vi "ma_SML Data Packing (real input).vi"(6 "reset?":bool, 8 "error in (no error)":errorcluster, 9 "%overlap":dbl format="%.2f", 10 "size":i32, 11 "x":dbl[](array[numeric]) format="%.2f") -> (0 "error out":errorcluster, 1 "data ready?":bool, 3 "y":dbl[](array[numeric]) format="%.2f")   [LabVIEW 2020, in "NI_MAPro.lvlib"]
uses:
  NI_MAPro.lvlib
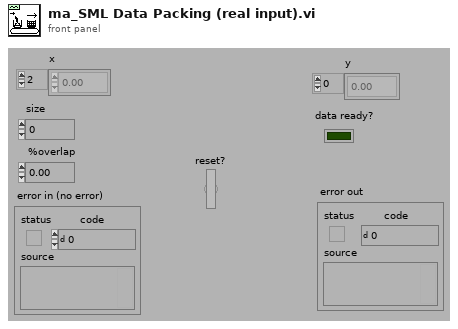
[diagram p1: front panel]
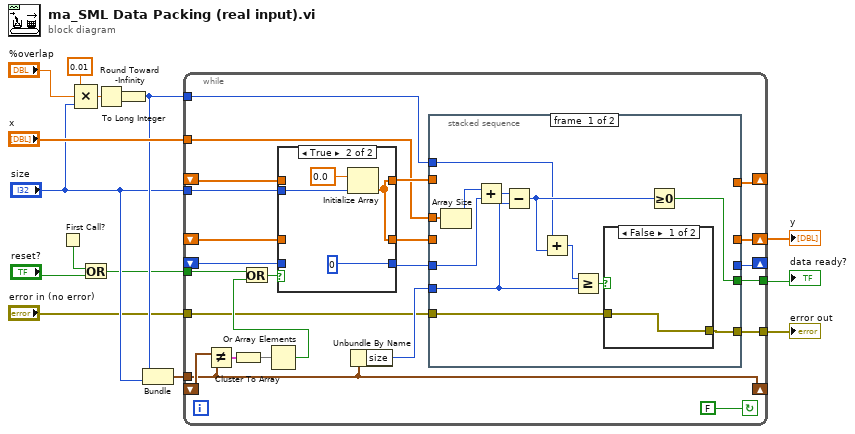
[diagram p0: block diagram]
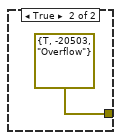
[diagram p2: hidden frame]
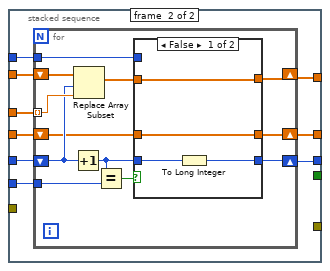
[diagram p3: hidden frame]
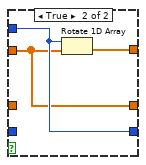
[diagram p4: hidden frame]
diagram:
  n1 = First Call?() -> (First Call?: T/F=w2:bool)
  n2 = Compound Arithmetic op=MULTIPLY(0.01, "%overlap", "size") -> (w15:dbl)
  n3 = Or(x=w2, y="reset?") -> (x .or. y?=w3:bool)
  n4 = Round Toward -Infinity(1:w15) -> (0:w12:dbl)
  n5 = To Long Integer(number=w12) -> (32bit integer=w9:i32)
  n6 = Bundle(w9, "size"="size") -> (w11:cluster{i32, "size":i32})  [unwired: 1 out]
  n7 = while {
    tunnel: "error in (no error)" -> [w16]
    tunnel: [w18] -> w4
    tunnel: w3 -> [w23]
    tunnel: [w24] -> w7
    tunnel: w9 -> [w25]
    tunnel: "x" -> [w30]
    tunnel: "size" -> [w34]
    shift-left: _ -> [w36]
    shift-right: [w26] -> _
    shift-left: _ -> [w35]
    shift-right: [w28] -> w6
    shift-left: _ -> [w33]
    shift-right: [w31] -> _
    tunnel: w11 -> [w20]
    shift-left: _ -> [w37]
    shift-right: [w20] -> _
    stop <- FALSE continue-if-true
    n8 = Not Equal?(x=w37, y=w20) -> (x != y?=w39:cluster{bool, "size":bool})
    n9 = Cluster To Array(cluster=w39) -> (array=w38:bool[])
    n10 = Or Array Elements(Boolean array=w38) -> (logical OR=w22:bool)
    n11 = Or(x=w23, y=w22) -> (x .or. y?=w21:bool)
    n12 = case shown="True" w21 {
      tunnel: [w84 0] -> w27
      tunnel: w36 -> [w84 _]
      tunnel: w35 -> [w83 _]
      tunnel: [w83 w85] -> w29
      tunnel: w34 -> [_ w86]
      tunnel: [w82 w85] -> w32
      tunnel: w33 -> [w82 _]
      frame False {
      }
      frame True {
        n13 = Initialize Array(0.0 ("Element Data"), w86) -> (w85:dbl[])
      }
    }
    n14 = Unbundle By Name(w20) -> ("size"=w19:i32)
    n15 = stacked-sequence {
      tunnel: w30 -> [w51 w62]
      tunnel: w32 -> [_ w57]
      tunnel: w27 -> [w41 w58]
      tunnel: w19 -> [w47 w61]
      tunnel: [_ w59] -> w26
      tunnel: [_ w54] -> w28
      tunnel: w29 -> [_ w55]
      tunnel: [_ w56] -> w31
      tunnel: w25 -> [w43 w60]
      tunnel: [w46 _] -> w24
      tunnel: [w48 _] -> w18
      tunnel: w16 -> [w40 _]
      frame #0 {
        n16 = Array Size(array=w51) -> (size(s)=w50:i32)
        n17 = Add(x=w50, y=w41) -> (x+y=w45:i32)
        n18 = Subtract(x=w45, y=w47) -> (x-y=w44:i32)
        n19 = Add(x=w43, y=w44) -> (x+y=w42:i32)
        n20 = Greater Or Equal?(x=w42, y=w47) -> (x >= y?=w49:bool)
        n21 = case shown="False" w49 {
          tunnel: [w52 errorcluster {"status"=TRUE, "code"=-20503, "source"="Overflow"} ("error out")] -> w48
          tunnel: w40 -> [w52 _]
          frame False {
          }
          frame True {
          }
        }
        n22 = Greater Or Equal To 0?(x=w44) -> (x >= 0?=w46:bool)
      }
      frame #1 {
        n23 = for {
          tunnel: w62 -> [w74] mode=indexing
          tunnel: w61 -> [w73]
          tunnel: w60 -> [w71]
          shift-right: [w66] -> w56
          shift-left: w57 -> [w67]
          shift-right: [w69] -> w59
          shift-left: w58 -> [w68]
          shift-right: [w63] -> w54
          shift-left: w55 -> [w64]
          n24 = Increment(x=w68) -> (x+1=w72:i32)
          n25 = Replace Array Subset(array=w67, new element=w74, index=w68) -> (w70:dbl[])
          n26 = Equal?(x=w72, y=w73) -> (x = y?=w65:bool)
          n27 = case shown="False" w65 {
            tunnel: w72 -> [w78 _]
            tunnel: [w77 w80] -> w69
            tunnel: [w76 w79] -> w63
            tunnel: w64 -> [w76 _]
            tunnel: w71 -> [_ w80]
            tunnel: w70 -> [w75 w79]
            tunnel: [w75 w81] -> w66
            frame False {
              n28 = To Long Integer(number=w78) -> (32bit integer=w77:i32)
            }
            frame True {
              n29 = Rotate 1D Array(1:w79, 2:w80) -> (0:w81:dbl[])
            }
          }
        }
      }
    }
  }
  "y" <- w6
  "data ready?" <- w7
  "error out" <- w4
